vi "VP_Owl1553_IMessageData_getMessageErrors.vi"(8 "error in (no error)":errorcluster, 11 "imessage data handle":u32) -> (0 "error out":errorcluster, 1 "error word":u32, 2 "DataErrorType":T1, 3 "imessage data handle":u32)   [LabVIEW 2013]
doc: "Get the errors for this message (if any). This is an OR'ed bitfield\nof @ref Owl1553DataErrorType.\n\n\nReturns:\nerrors for the message, @ref OWL1553_DATA_ERROR_NONE if\nthere are none"
uses:
  Program Files (x86)/National Instruments/LabVIEW 2013/user.lib/MIL-STD-1553/Owl1553.lvlib
  owl1553.dll
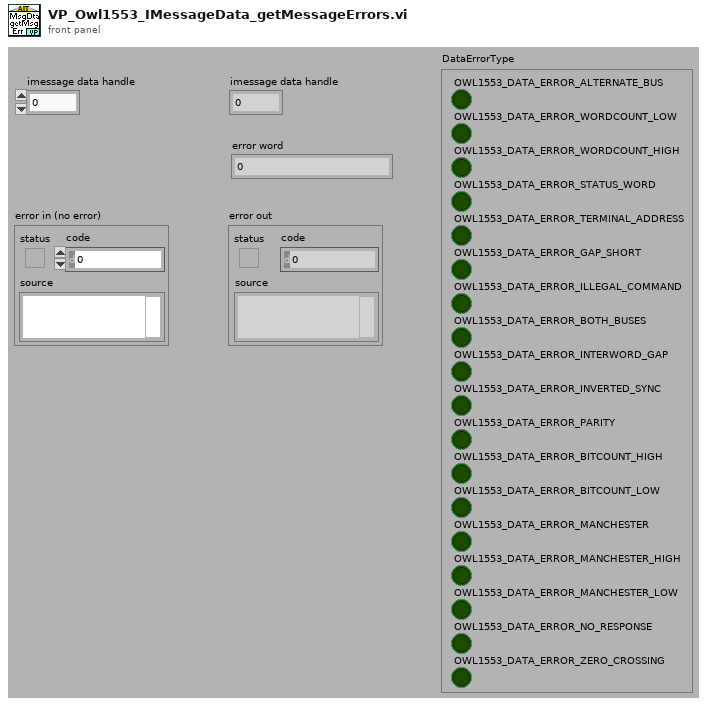
[diagram p1: front panel]
types:
  T1 = cluster{"OWL1553_DATA_ERROR_ALTERNATE_BUS":bool, "OWL1553_DATA_ERROR_WORDCOUNT_LOW":bool, "OWL1553_DATA_ERROR_WORDCOUNT_HIGH":bool, "OWL1553_DATA_ERROR_STATUS_WORD":bool, "OWL1553_DATA_ERROR_TERMINAL_ADDRESS":bool, "OWL1553_DATA_ERROR_GAP_SHORT":bool, "OWL1553_DATA_ERROR_ILLEGAL_COMMAND":bool, "OWL1553_DATA_ERROR_BOTH_BUSES":bool, "OWL1553_DATA_ERROR_INTERWORD_GAP":bool, "OWL1553_DATA_ERROR_INVERTED_SYNC":bool, "OWL1553_DATA_ERROR_PARITY":bool, "OWL1553_DATA_ERROR_BITCOUNT_HIGH":bool, "OWL1553_DATA_ERROR_BITCOUNT_LOW":bool, "OWL1553_DATA_ERROR_MANCHESTER":bool, "OWL1553_DATA_ERROR_MANCHESTER_HIGH":bool, "OWL1553_DATA_ERROR_MANCHESTER_LOW":bool, "OWL1553_DATA_ERROR_NO_RESPONSE":bool, "OWL1553_DATA_ERROR_ZERO_CROSSING":bool}
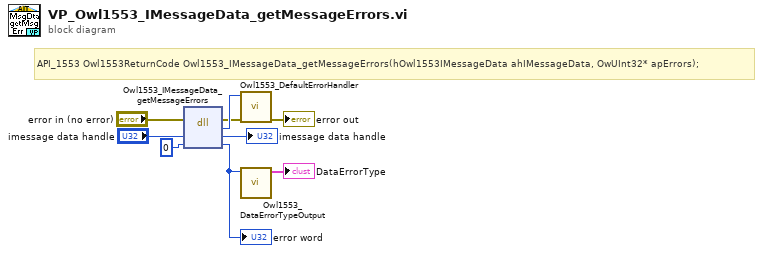
[diagram p0: block diagram]
diagram:
  # "API_1553 Owl1553ReturnCode Owl1553_IMessageData_getMessageErrors(hOwl1553IMessageData ahIMessageData, OwUInt32* apErrors);"
  n1 = dll-call lib="owl1553.*" fn="Owl1553_IMessageData_getMessageErrors"(error in="error in (no error)", "imessage data handle"="imessage data handle", "errors"=u32 0) -> (error out=w6:errorcluster, "return type"=w7:i32, "imessage data handle"=→"imessage data handle":u32, "errors"=w1:u32)  [unwired: 2 in, 1 out]
  "error word" <- w1
  n2 = call "Owl1553_DefaultErrorHandler.vi"("error in (no error)"=w6, "error code"=w7) -> ("error out"=→"error out":errorcluster)  [unwired: 9 in]
  n3 = call "Owl1553_DataErrorTypeOutput.vi"("error type"=w1) -> ("DataErrorType"=→"DataErrorType":T1)  [unwired: 10 in]
